vi "veristandSteps-assemblyProjectFile-getDotNetProjectHintPaths.vi"(8 "error in":errorcluster, 10 "Parameters":string[](array[string]), 11 "CLI in":refnum<class "CLI.lvclass">) -> (0 "error out":errorcluster, 1 "New Assembly Include Paths":string[](array[string]), 2 "New Assembly Hint Paths":string[](array[string]), 3 "CLI out":refnum<class "CLI.lvclass">)   [LabVIEW 2014, in "veristand-steps-build-system.lvlib"]
uses:
  <vilib>/Wiresmith Technology/LabVIEW CLI/CLI Class/CLI.lvclass
  veristand-steps-build-system.lvlib
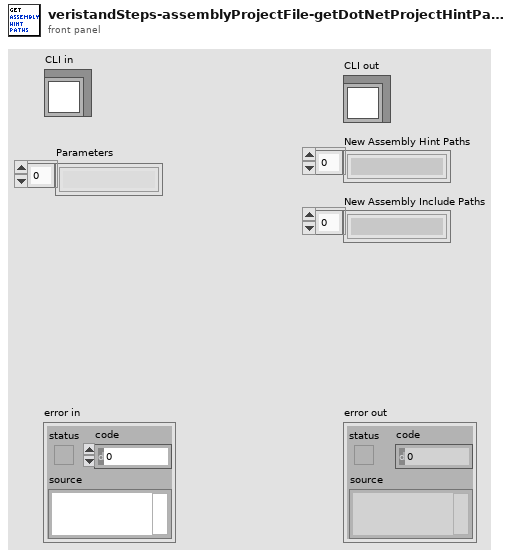
[diagram p1: front panel]
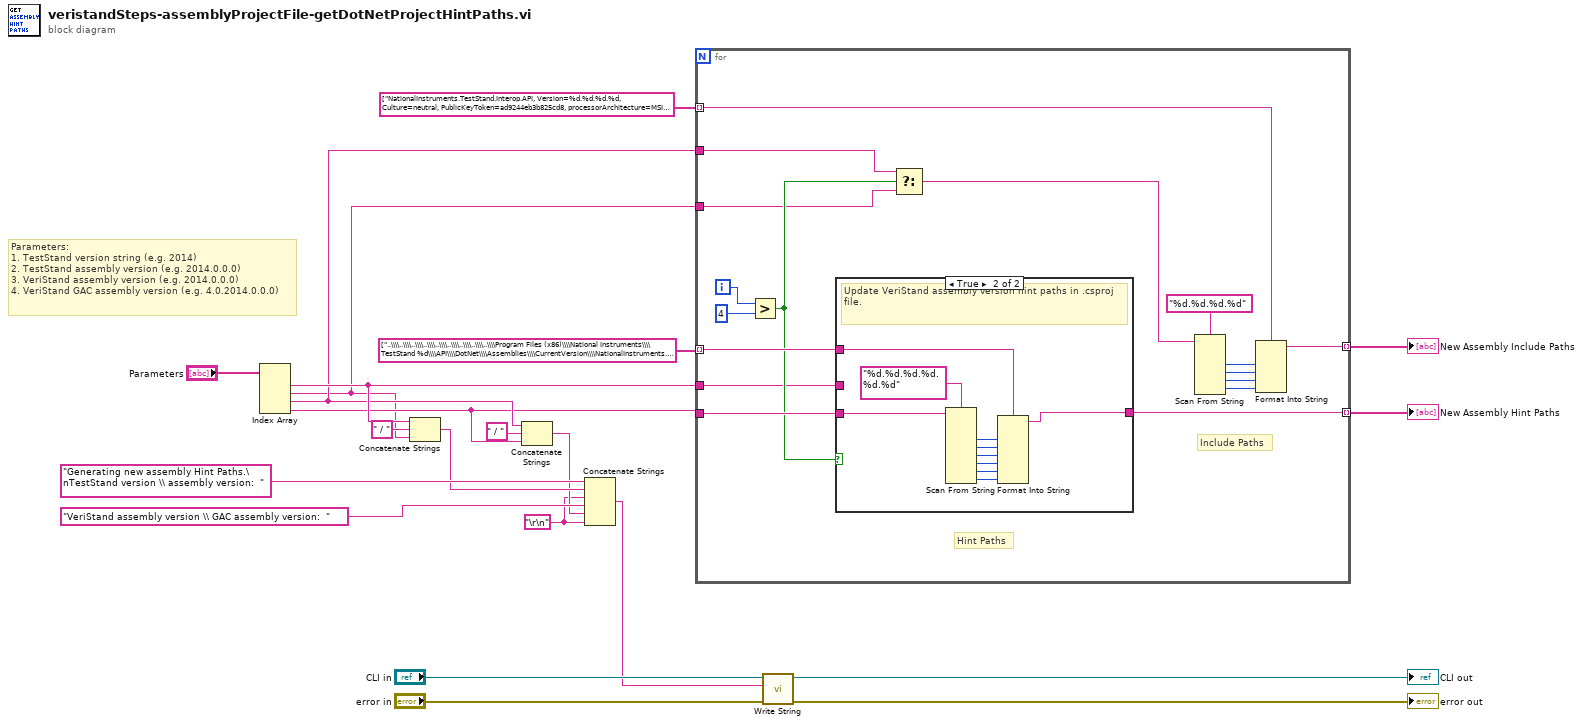
[diagram p0: block diagram]
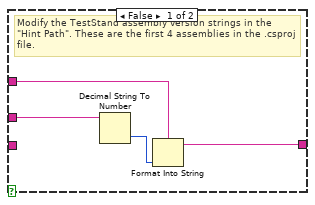
[diagram p2: hidden frame]
diagram:
  w6 = "\r\n"
  # "Parameters:\n1. TestStand version string (e.g. 2014)\n2. TestStand assembly version (e.g. 2014.0.0.0) \n3. VeriStand assembly version (e.g. 2014.0.0.0)\n4. VeriStand GAC assembly version (e.g. 4.0.2014.0.0.0)"
  n1 = Index Array(array="Parameters") -> (element #1=w12:string, element #2=w3:string, element #3=w8:string, element #4=w4:string)  [unwired: 4 in]
  n2 = Concatenate Strings(w12, " / " ("string"), w3) -> (w10:string)
  n3 = Concatenate Strings(w8, " / " ("string"), w4) -> (w7:string)
  n4 = Concatenate Strings("Generating new assembly Hint Paths.\nTestStand version \\ assembly version:  ", w10, w6, "VeriStand assembly version \\ GAC assembly version:  ", w7, w6) -> (w5:string)
  n5 = for {
    tunnel: [w34] -> w16 mode=indexing
    tunnel: string[] ["..\\\\..\\\\..\\\\..\\\\..\\\\..\\\\..\\\\..\\\\..\\\\Program Files (x86)\\\\National Instruments\\\\TestStand %d\\\\API\\\\DotNet\\\\Assemblies\\\\CurrentVersion\\\\NationalInstruments.TestStand.Interop.API.dll", "..\\\\..\\\\..\\\\..\\\\..\\\\..\\\\..\\\\..\\\\..\\\\Program Files (x86)\\\\National Instruments\\\\TestStand %d\\\\API\\\\DotNet\\\\Assemblies\\\\CurrentVersion\\\\NationalInstruments.TestStand.Interop.UI.dll", "..\\\\..\\\\..\\\\..\\\\..\\\\..\\\\..\\\\..\\\\..\\\\Program Files (x86)\\\\National Instruments\\\\TestStand %d\\\\API\\\\DotNet\\\\Assemblies\\\\CurrentVersion\\\\NationalInstruments.TestStand.Interop.UI.AxControls.dll", "..\\\\..\\\\..\\\\..\\\\..\\\\..\\\\..\\\\..\\\\..\\\\Program Files (x86)\\\\National Instruments\\\\TestStand %d\\\\API\\\\DotNet\\\\Assemblies\\\\CurrentVersion\\\\NationalInstruments.TestStand.Interop.UISupport.dll", "..\\\\..\\\\..\\\\..\\\\..\\\\..\\\\..\\\\..\\\\..\\\\Program Files (x86)\\\\National Instruments\\\\TestStand %d\\\\Bin\\\\NationalInstruments.TestStand.Utility.dll", "..\\\\..\\\\..\\\\..\\\\..\\\\..\\\\..\\\\..\\\\Windows\\\\Microsoft.NET\\\\assembly\\\\GAC_MSIL\\\\NationalInstruments.VeriStand\\\\v%d.%d_%d.%d.%d.%d__a6d690c380daa308\\\\NationalInstruments.VeriStand.dll", "..\\\\..\\\\..\\\\..\\\\..\\\\..\\\\..\\\\..\\\\Windows\\\\Microsoft.NET\\\\assembly\\\\GAC_MSIL\\\\NationalInstruments.VeriStand.ClientAPI\\\\v%d.%d_%d.%d.%d.%d__a6d690c380daa308\\\\NationalInstruments.VeriStand.ClientAPI.dll", "..\\\\..\\\\..\\\\..\\\\..\\\\..\\\\..\\\\..\\\\Windows\\\\Microsoft.NET\\\\assembly\\\\GAC_MSIL\\\\NationalInstruments.VeriStand.DataTypes\\\\v%d.%d_%d.%d.%d.%d__a6d690c380daa308\\\\NationalInstruments.VeriStand.DataTypes.dll", "..\\\\..\\\\..\\\\..\\\\..\\\\..\\\\..\\\\..\\\\Windows\\\\Microsoft.NET\\\\assembly\\\\GAC_MSIL\\\\NationalInstruments.VeriStand.RealTimeSequenceDefinitionAPI\\\\v%d.%d_%d.%d.%d.%d__a6d690c380daa308\\\\NationalInstruments.VeriStand.RealTimeSequenceDefinitionAPI.dll", "..\\\\..\\\\..\\\\..\\\\..\\\\..\\\\..\\\\..\\\\Windows\\\\Microsoft.NET\\\\assembly\\\\GAC_MSIL\\\\NationalInstruments.VeriStand.SystemDefinitionAPI\\\\v%d.%d_%d.%d.%d.%d__a6d690c380daa308\\\\NationalInstruments.VeriStand.SystemDefinitionAPI.dll", "..\\\\..\\\\..\\\\..\\\\..\\\\..\\\\..\\\\..\\\\Windows\\\\Microsoft.NET\\\\assembly\\\\GAC_MSIL\\\\NationalInstruments.VeriStand.SystemStorage\\\\v%d.%d_%d.%d.%d.%d__a6d690c380daa308\\\\NationalInstruments.VeriStand.SystemStorage.dll", "..\\\\..\\\\..\\\\..\\\\..\\\\..\\\\..\\\\..\\\\Windows\\\\Microsoft.NET\\\\assembly\\\\GAC_MSIL\\\\NationalInstruments.VeriStand.SystemStorageUI\\\\v%d.%d_%d.%d.%d.%d__a6d690c380daa308\\\\NationalInstruments.VeriStand.SystemStorageUI.dll", "..\\\\..\\\\..\\\\..\\\\..\\\\..\\\\..\\\\..\\\\Windows\\\\Microsoft.NET\\\\assembly\\\\GAC_MSIL\\\\NationalInstruments.VeriStand.WorkspaceMacro\\\\v%d.%d_%d.%d.%d.%d__a6d690c380daa308\\\\NationalInstruments.VeriStand.WorkspaceMacro.dll"] -> [w33] mode=indexing
    tunnel: [w32] -> w15 mode=indexing
    tunnel: w4 -> [w30]
    tunnel: w8 -> [w28]
    tunnel: w12 -> [w23]
    tunnel: string[] ["NationalInstruments.TestStand.Interop.API, Version=%d.%d.%d.%d, Culture=neutral, PublicKeyToken=ad9244eb3b825cd8, processorArchitecture=MSIL", "NationalInstruments.TestStand.Interop.UI, Version=%d.%d.%d.%d, Culture=neutral, PublicKeyToken=ad9244eb3b825cd8, processorArchitecture=MSIL", "NationalInstruments.TestStand.Interop.UI.AxControls, Version=%d.%d.%d.%d, Culture=neutral, PublicKeyToken=ad9244eb3b825cd8, processorArchitecture=MSIL", "NationalInstruments.TestStand.Interop.UI.Support, Version=%d.%d.%d.%d, Culture=neutral, PublicKeyToken=ad9244eb3b825cd8, processorArchitecture=MSIL", "NationalInstruments.TestStand.Interop.Utility, Version=%d.%d.%d.%d, Culture=neutral, processorArchitecture=x86", "NationalInstruments.VeriStand, Version=%d.%d.%d.%d, Culture=neutral, PublicKeyToken=a6d690c380daa308, processorArchitecture=MSIL", "NationalInstruments.VeriStand.ClientAPI, Version=%d.%d.%d.%d, Culture=neutral, PublicKeyToken=a6d690c380daa308, processorArchitecture=MSIL", "NationalInstruments.VeriStand.DataTypes, Version=%d.%d.%d.%d, Culture=neutral, PublicKeyToken=a6d690c380daa308, processorArchitecture=MSIL", "NationalInstruments.VeriStand.RealTimeSequenceDefinitionApi, Version=%d.%d.%d.%d, Culture=neutral, PublicKeyToken=a6d690c380daa308, processorArchitecture=MSIL", "NationalInstruments.VeriStand.SystemDefinitionAPI, Version=%d.%d.%d.%d, Culture=neutral, PublicKeyToken=a6d690c380daa308, processorArchitecture=MSIL", "NationalInstruments.VeriStand.SystemStorage, Version=%d.%d.%d.%d, Culture=neutral, PublicKeyToken=a6d690c380daa308, processorArchitecture=MSIL", "NationalInstruments.VeriStand.SystemStorageUI, Version=%d.%d.%d.%d, Culture=neutral, PublicKeyToken=a6d690c380daa308, processorArchitecture=MSIL", "NationalInstruments.VeriStand.WorkspaceMacro, Version=%d.%d.%d.%d, Culture=neutral, PublicKeyToken=a6d690c380daa308, processorArchitecture=MSIL"] -> [w25] mode=indexing
    tunnel: w3 -> [w22]
    i -> [w31]
    # "Hint Paths"
    # "Include Paths"
    n6 = Greater?(x=w31, y=4 ("x")) -> (0:w29:bool)
    n7 = case shown="True" w29 {
      tunnel: w33 -> [w42 w52]
      tunnel: [w41 w51] -> w32
      tunnel: w30 -> [_ w50]
      tunnel: w23 -> [w39 _]
      frame False {
        # "Modify the TestStand assembly version strings in the \"Hint Path\". These are the first 4 assemblies in the .csproj file."
        n8 = Decimal String To Number(string=w39) -> (number=w40:i32)  [unwired: 2 in, 1 out]
        n9 = Format Into String(format string=w42, w40) -> (resulting string=w41:string)  [unwired: 2 in, 1 out]
      }
      frame True {
        # "Update VeriStand assembly version hint paths in .csproj file."
        n10 = Scan From String(format string="%d.%d.%d.%d.%d.%d", input string=w50) -> (output 1=w49:i32, output 2=w48:i32, output 3=w47:i32, output 4=w46:i32, output 5=w45:i32, output 6=w44:i32)  [unwired: 8 in, 3 out]
        n11 = Format Into String(format string=w52, w49, w48, w47, w46, w45, w44) -> (resulting string=w51:string)  [unwired: 2 in, 1 out]
      }
    }
    n12 = Select(t=w28, s=w29, f=w22) -> (s? t:f=w27:string)
    n13 = Scan From String(format string="%d.%d.%d.%d", input string=w27) -> (output 1=w38:i32, output 2=w37:i32, output 3=w36:i32, output 4=w35:i32)  [unwired: 6 in, 3 out]
    n14 = Format Into String(format string=w25, w38, w37, w36, w35) -> (resulting string=w34:string)  [unwired: 2 in, 1 out]
  }
  "New Assembly Include Paths" <- w16
  "New Assembly Hint Paths" <- w15
  n15 = call <vilib>:"Write String.vi"("error in (no error)"="error in", "Text to Write"=w5, "CLI in"="CLI in") -> ("error out"=→"error out":errorcluster, "CLI out"=→"CLI out":refnum<class "CLI.lvclass">)  [unwired: 7 in]
